vi "Set Elapsed Time (seconds).vi"(8 "error in (no error)":errorcluster, 10 "Elapsed Time (seconds)":dbl, 11 "Timer in":refnum<class "Timer.lvclass">) -> (0 "error out":errorcluster, 3 "Timer out":refnum<class "Timer.lvclass">)   [LabVIEW 2018, in "Timer.lvclass"]
uses:
  Timer.lvclass
  Timer.lvclass/Timer.ctl
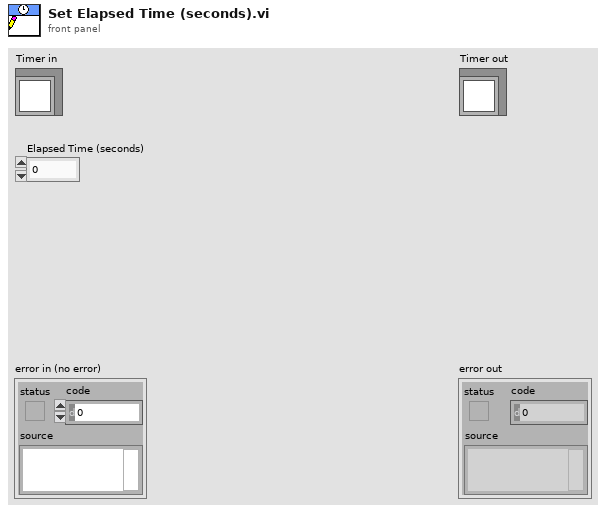
[diagram p1: front panel]
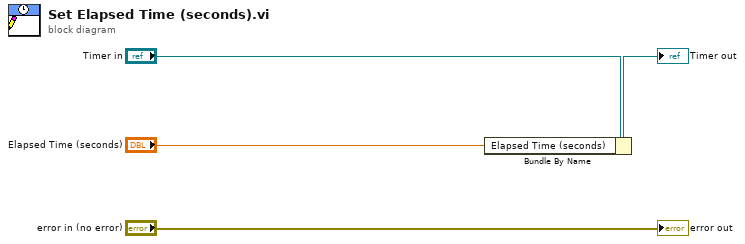
[diagram p0: block diagram]
diagram:
  n1 = Bundle By Name(cluster="Timer in", "Elapsed Time (seconds)"="Elapsed Time (seconds)") -> (→"Timer out":refnum<class "Timer.lvclass">)
  "error out" <- "error in (no error)"
